vi "Set_Needle_Valve.vi"   [LabVIEW 2016]
uses:
  Global Variables/global.vi
  Instrument_Setup.vi
types:
  T1 = typedef "ITCIO.ctl" = cluster{"Address":T2, "Version":T3, "Ch 1 dec places":i16, "Ch 2 dec places":i16, "Ch 3 dec places":i16, "Ch1 Name":string, "Ch2 Name":string, "Ch3 Name":string}
  T2 = typedef "OxfordAddress.ctl" = cluster{"Com Port":i32, "ISOBUS Address":i32, "GPIB Address":i16, "Communication":enum16{"RS232", "ISOBUS", "GPIB", "Gateway"}}
  T3 = typedef "ITCVersion.ctl" = enum16{"ITC502", "ITC503", "ITC601"}
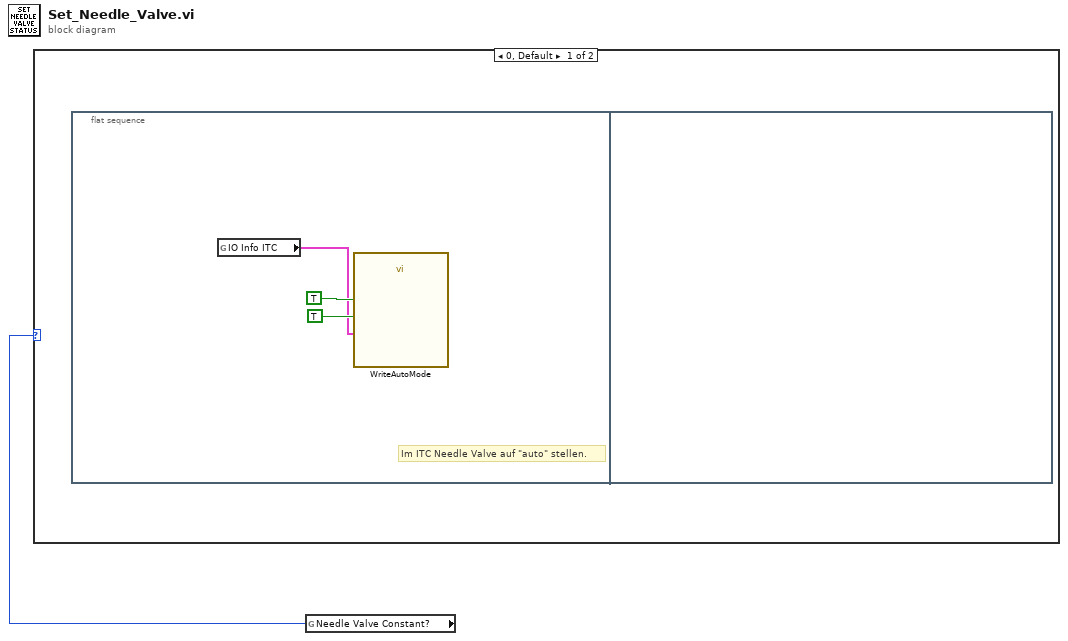
[diagram p0: block diagram]
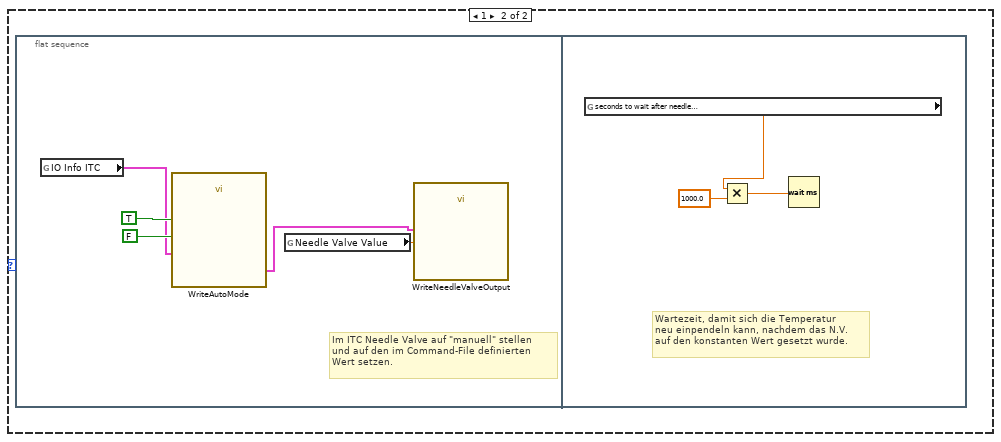
[diagram p2: hidden frame]
diagram:
  n1 = global read "global.vi" "Needle Valve Constant?"() -> (w1:i32)
  n2 = case shown="0, Default" w1 {
    frame 0, Default {
      n3 = flat-sequence {
        frame #0 {
          # "Im ITC Needle Valve auf \"auto\" stellen."
          n4 = global read "Instrument_Setup.vi" "IO Info ITC"() -> (w2:T1)
          n5 = call "WriteAutoMode.vi"("Auto Needle Valve"=TRUE, "Auto Heat"=TRUE, "ITC IO Info"=w2) -> ()  [unwired: 1 out]
        }
        frame #1 {
        }
      }
    }
    frame 1 {
      n6 = flat-sequence {
        frame #0 {
          # "Im ITC Needle Valve auf \"manuell\" stellen\nund auf den im Command-File definierten\nWert setzen."
          n7 = global read "Instrument_Setup.vi" "IO Info ITC"() -> (w5:T1)
          n8 = call "WriteAutoMode.vi"("Auto Needle Valve"=FALSE, "Auto Heat"=TRUE, "ITC IO Info"=w5) -> ("ITC IO Info"=w6:T1)
          n9 = global read "global.vi" "Needle Valve Value"() -> (w7:dbl)
          n10 = call "WriteNeedleValveOutput.vi"("Needle Valve Output (%"=w7, "ITC IO Info"=w6) -> ()  [unwired: 1 in, 1 out]
        }
        frame #1 {
          # "Wartezeit, damit sich die Temperatur\nneu einpendeln kann, nachdem das N.V.\nauf den konstanten Wert gesetzt wurde."
          n11 = global read "Instrument_Setup.vi" "seconds to wait after needle\nvalve was set from auto to\nmanual"() -> (w11:dbl)
          n12 = Multiply(x=w11, y=1000.0) -> (x*y=w10:dbl)
          n13 = Wait (ms)(milliseconds to wait=w10) -> ()  [unwired: 1 out]
        }
      }
    }
  }
